vi "Instrumento_caracterizacion_4.vi"() -> ()   [LabVIEW 2013]
uses:
  <vilib>/Analysis/NI_AALBase.lvlib
panel:
  in  "Tab Control":enum32{"Live Picture", "ICImagingControl"}(tab)
  out "Live Picture":picture
  in  "ICImagingControl":refnum<k7>(container)
  in  "Pasos por vuelta\nM1(746)          M2(646)      M3(740)       M4(766)":dbl[](array[numeric])
  in  "Nombre de archivo 2":string="In"
  out "a":bool
  out "Angulo actual":dbl[](array[numeric])
  in  "Ejecutar desde txt":bool
  in  "Txt con medidas a realizar":path=path "C:/Users/franjas/Documents/rutinas-calibracion-slm/measures.txt"
  in  "Camino a ArduinoSteeper.py":path=path "C:/Users/franjas/Documents/rutinas-calibracion-slm"
  in  "Directorio scripts matlab 2":path=path "C:/Users/franjas/Documents/rutinas-calibracion-slm"
  out "o":bool
  in  "Nombre de archivo":string="In1"
  in  "Start":bool
  in  "Seleción método":bool
  in  "Ángulos de elementos ópticos:\nL2_in        L4_in     L4_out  P__out":dbl[](array[numeric])=[0.0, 0.0, 0.0, 0.0]
  in  "Shutter":bool
  in  "Stop VI":bool
  in  "Amp vs ng":bool
  in  "fas vs ng":bool
  in  "Configurar para franjas":bool
  in  "Exit live":bool
  in  "ContinuousCapture":bool
  in  "File to load":path
  in  "File to save":path
  in  "VCD Properties":bool
  in  "Save properties":bool
  in  "Load properties":bool
  out "Video formats":string[](array[string])
  out "Devices":string[](array[string])
  out "Histogram Graph":T1(graph)
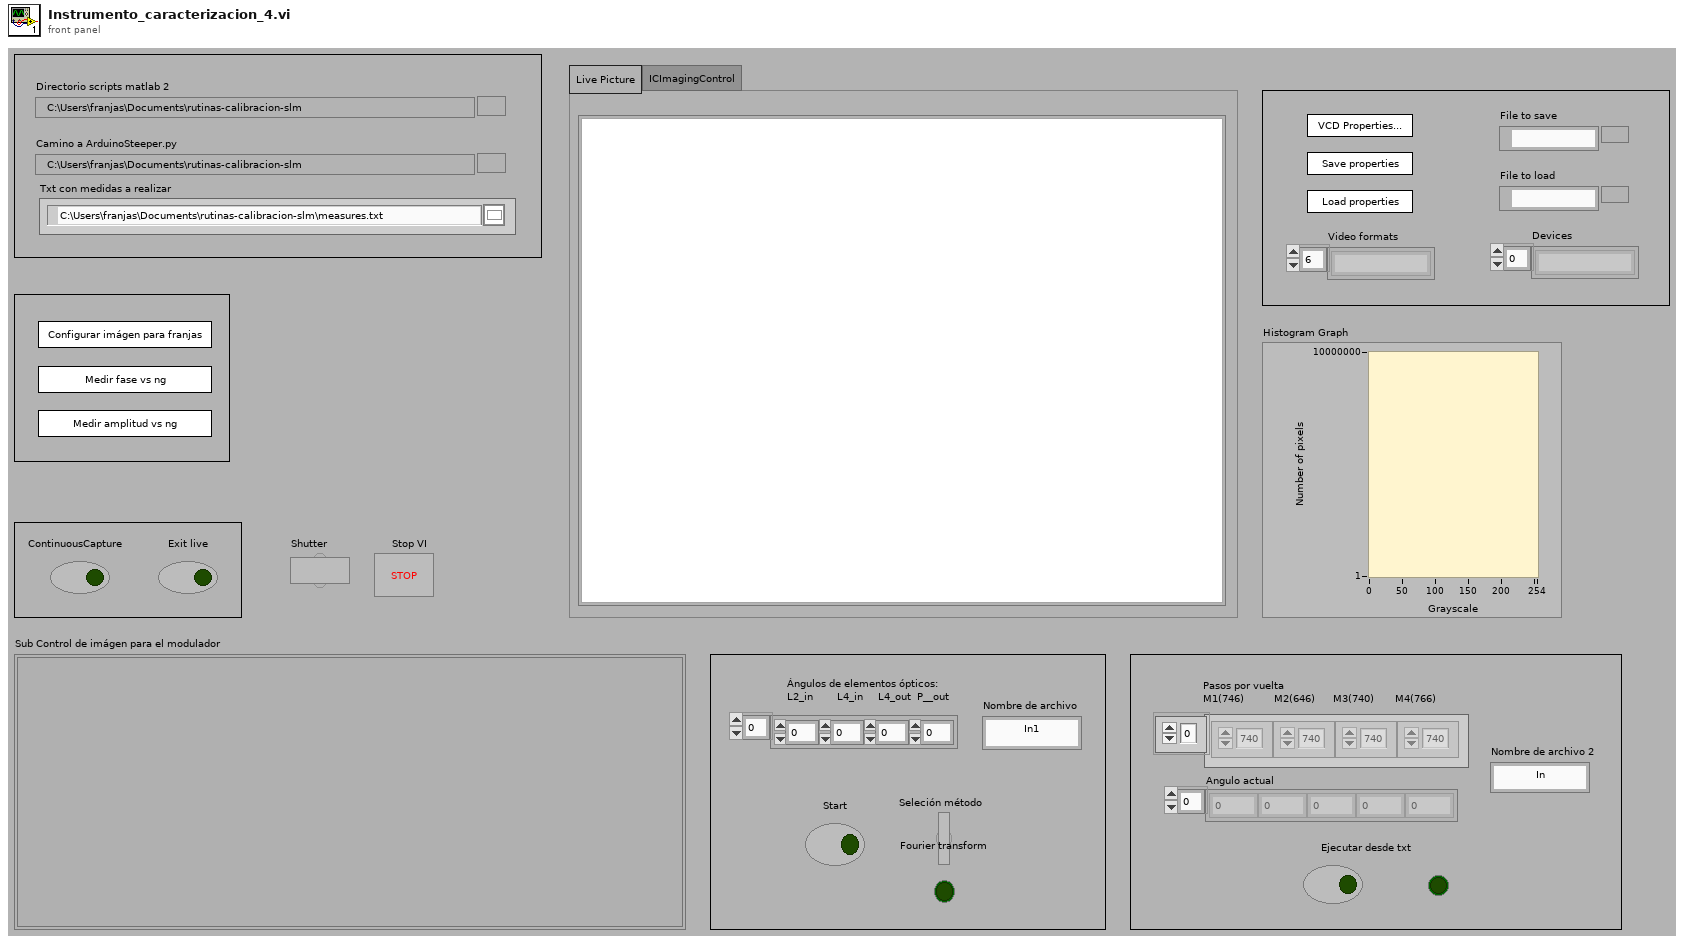
[diagram p1: front panel]
types:
  T1 = cluster{"X Values":dbl[], "Histogram: h(x)":i32[]}
  T2 = typedef "imagedata.ctl" = cluster{"image type":i32, "image depth":i32, "image":u8[], "mask":u8[], "colors":u32[], "Rectangle":cluster{"left":i16, "top":i16, "right":i16, "bottom":i16}}
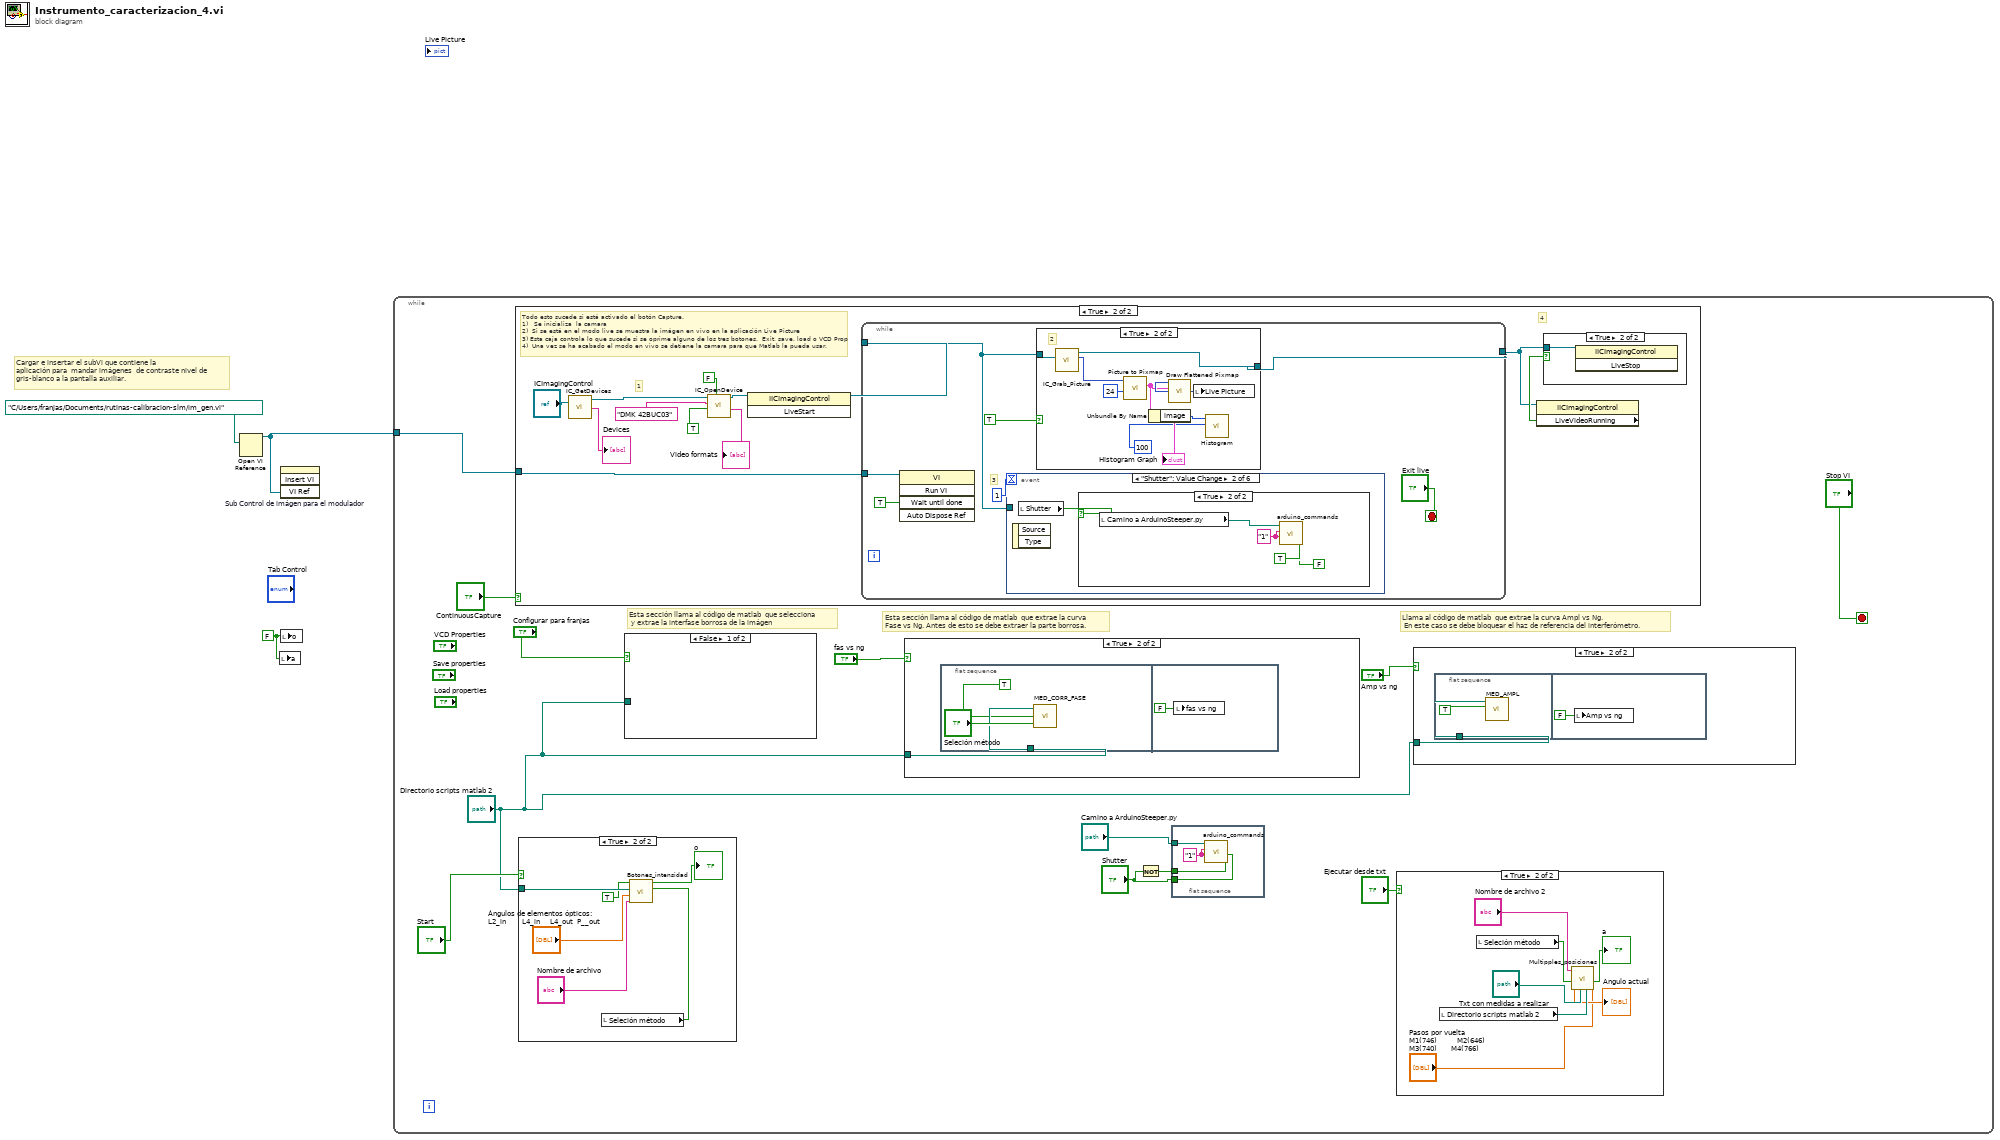
[diagram p0: block diagram]
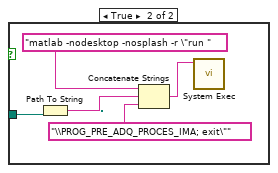
[diagram p6: hidden frame]
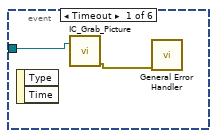
[diagram p8: hidden frame]
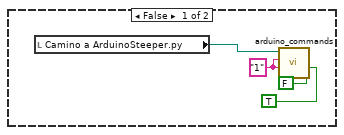
[diagram p9: hidden frame]
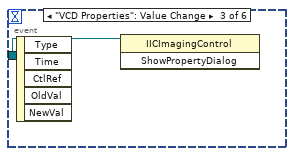
[diagram p10: hidden frame]
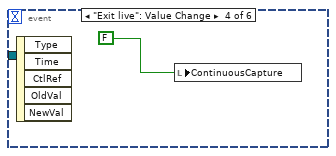
[diagram p11: hidden frame]
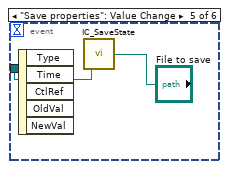
[diagram p12: hidden frame]
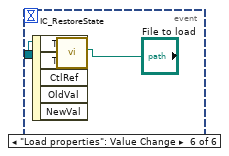
[diagram p13: hidden frame]
diagram:
  w1 = FALSE ("o")
  # "Cargar e insertar el subVi que contiene la \naplicación para  mandar imágenes  de contraste nivel de gris-blanco a la pantalla auxiliar."
  n1 = Open VI Reference(vi path=path "C:/Users/franjas/Documents/rutinas-calibracion-slm/im_gen.vi") -> (vi reference=w2:refnum<vi>)  [unwired: 5 in, 1 out]
  n2 = local write "a"(w1) -> ()
  n3 = invoke on="Sub Control de imágen para el modulador" class="SubPanel" method="Insert VI"("VI Ref"=w2) -> ()  [unwired: 3 in, 4 out]
  n4 = local write "o"(w1) -> ()
  n5 = while {
    tunnel: w2 -> [w13]
    stop <- "Stop VI" stop-if-true
    # "Llama al código de matlab  que extrae la curva Ampl vs Ng.\n En este caso se debe bloquear el haz de referencia del interferómetro."
    # "Esta sección llama al código de matlab  que extrae la curva\nFase vs Ng. Antes de esto se debe extraer la parte borrosa."
    # "Esta sección llama al código de matlab  que selecciona\n y extrae la interfase borrosa de la imágen"
    n6 = case shown="True" "ContinuousCapture" {
      tunnel: w13 -> [_ w47]
      frame False {
      }
      frame True {
        # "4"
        # "1"
        # "Todo esto sucede si está activado el botón Capture.  \n1)   Se inicializa  la camara \n2)  Si se está en el modo live se muestra la imágen en vivo en la aplicación Live Picture\n3) Esta caja controla lo que sucede si se oprime alguno de los tres botones,  Exit, save, load o VCD Prop\n4)  Una vez se ha acabado el modo en vivo se detiene la camara para que Matlab la pueda usar."
        n7 = call <userlib>:"IC_GetDevices.vi"("ICImagingControl In"="ICImagingControl") -> ("ICImagingControl Out"=w56:refnum<k7>, "Devices"=→"Devices":string[])  [unwired: 1 in, 1 out]
        n8 = call <userlib>:"IC_OpenDevice.vi"("Color"=FALSE, "Live"=TRUE, "Device"="DMK 42BUC03", "ICImagingControl In"=w56) -> ("VideoFormats"=→"Video formats":string[], "ICImagingControl Out"=w50:refnum<k7>)  [unwired: 2 in, 4 out]
        n9 = invoke class="IICImagingControl" method="LiveStart"(reference=w50) -> (reference out=w48:refnum<k7>)  [unwired: 2 in, 2 out]
        n10 = while {
          tunnel: w48 -> [w62]
          tunnel: [w65] -> w49
          tunnel: w47 -> [w64]
          stop <- "Exit live" stop-if-true
          # "3"
          n11 = invoke class="VI" method="Run VI"(reference=w64, "Wait until done"=TRUE ("Wait Until Done")) -> ()  [unwired: 3 in, 5 out]
          n12 = event shown="[1] \"Shutter\": Value Change" {
            selector: _ -> [_ _ _ _ _ _]
            dyn-events: _ -> [_ _ _ _ _ _]
            timeout: 1 -> [_ _ _ _ _ _]
            tunnel: w62 -> [w66 _ w77 _ w80 w82]
            event Timeout {
              n13 = event-data() -> ()  [unwired: 1 in, 2 out]
              n14 = call <userlib>:"IC_Grab_Picture.vi"("ICImagingControl In"=w66) -> ("Error Out"=w67:errorcluster)  [unwired: 1 in, 3 out]
              n15 = call <vilib>:"General Error Handler.vi"("error in (no error)"=w67) -> ()  [unwired: 10 in, 5 out]
            }
            event "Shutter": Value Change {
              n16 = event-data() -> ()  [unwired: 1 in, 2 out]
              n17 = local read "Shutter"() -> (w68:bool)
              n18 = case shown="True" w68 {
                frame False {
                  w71 = "1" ("Argumento")
                  n19 = local read "Camino a ArduinoSteeper.py"() -> (w72:path)
                  n20 = call "arduino_commands.vi"("Shutter off"=FALSE, "Shutter on"=TRUE ("Shutter off"), "Argumento"=w71, "Número de motor"=w71, "Directorio scripts ArduinoStepper.py"=w72) -> ()  [unwired: 6 in, 1 out]
                }
                frame True {
                  w75 = "1" ("Argumento")
                  n21 = local read "Camino a ArduinoSteeper.py"() -> (w76:path)
                  n22 = call "arduino_commands.vi"("Shutter off"=TRUE, "Shutter on"=FALSE, "Argumento"=w75, "Número de motor"=w75, "Directorio scripts ArduinoStepper.py"=w76) -> ()  [unwired: 6 in, 1 out]
                }
              }
            }
            event "VCD Properties": Value Change {
              n23 = event-data() -> ()  [unwired: 1 in, 5 out]
              n24 = invoke class="IICImagingControl" method="ShowPropertyDialog"(reference=w77) -> ()  [unwired: 2 in, 3 out]
            }
            event "Exit live": Value Change {
              n25 = event-data() -> ()  [unwired: 1 in, 5 out]
              n26 = local write "ContinuousCapture"(FALSE ("CApture")) -> ()
            }
            event "Save properties": Value Change {
              n27 = event-data() -> ()  [unwired: 1 in, 5 out]
              n28 = call <userlib>:"IC_SaveState.vi"("file path"="File to save", "ICImagingControl In"=w80) -> ()  [unwired: 1 in, 2 out]
            }
            event "Load properties": Value Change {
              n29 = event-data() -> ()  [unwired: 1 in, 5 out]
              n30 = call <userlib>:"IC_RestoreState.vi"("File Path"="File to load", "ICImagingControl"=w82) -> ()  [unwired: 2 in, 2 out]
            }
          }
          n31 = case shown="True" TRUE {
            tunnel: w62 -> [w83 w89]
            tunnel: [w83 w84] -> w65
            frame False {
            }
            frame True {
              # "2"
              n32 = call <userlib>:"IC_Grab_Picture.vi"("ICImagingControl In"=w89) -> ("ICImagingControl Out"=w84:refnum<k7>, "Picture Out"=w92:picture)  [unwired: 1 in, 2 out]
              n33 = call <vilib>:"Picture to Pixmap.vi"("depth"=24, "picture"=w92) -> ("image data"=w88:T2)  [unwired: 8 in, 1 out]
              n34 = Unbundle By Name(w88) -> ("image"=w87:u8[])
              n35 = call <vilib>:"Draw Flattened Pixmap.vi"("image data"=w88) -> ("new picture"=w90:picture)  [unwired: 8 in]
              n36 = local write "Live Picture"(w90) -> ()
              n37 = call <vilib>:"Histogram.vi"("intervals"=100, "X"=w87) -> ("Histogram Graph"=→"Histogram Graph":T1)  [unwired: 6 in, 3 out]
            }
          }
        }
        n38 = property class="IICImagingControl"(reference=w49) -> ("LiveVideoRunning"=w51:bool)  [unwired: 1 in, 2 out]
        n39 = case shown="True" w51 {
          tunnel: w49 -> [_ w93]
          frame False {
          }
          frame True {
            n40 = invoke class="IICImagingControl" method="LiveStop"(reference=w93) -> ()  [unwired: 2 in, 3 out]
          }
        }
      }
    }
    n41 = case shown="True" "Start" {
      tunnel: "Directorio scripts matlab 2" -> [_ w32]
      frame False {
      }
      frame True {
        n42 = local read "Seleción método"() -> (w29:bool)
        n43 = call "Botones_intensidad.vi"("Seleción método"=w29, "String"="Nombre de archivo", "Array"="Ángulos de elementos ópticos:\nL2_in        L4_in     L4_out  P__out", "Directorio scripts matlab 2"=w32, "I1"=TRUE) -> (3:→"o":bool)  [unwired: 6 in]
      }
    }
    n44 = case shown="False" "Configurar para franjas" {
      tunnel: "Directorio scripts matlab 2" -> [_ w42]
      frame False {
      }
      frame True {
        n45 = Path To String(path=w42) -> (string=w46:string)
        n46 = Concatenate Strings("matlab -nodesktop -nosplash -r \"run " ("command line"), w46, "\\PROG_PRE_ADQ_PROCES_IMA; exit\"" ("command line")) -> (w45:string)
        n47 = call <vilib>:"System Exec.vi"("command line"=w45) -> ()  [unwired: 7 in, 4 out]
      }
    }
    n48 = case shown="True" "fas vs ng" {
      tunnel: "Directorio scripts matlab 2" -> [_ w37]
      frame False {
      }
      frame True {
        n49 = flat-sequence {
          tunnel: w37 -> [w39]
          frame #0 {
            n50 = call "MED_CORR_FASE.vi"("Seleción método"="Seleción método", "Ejecucion"=TRUE ("Boolean"), "Directorio scripts matlab"=w39) -> ()
          }
          frame #1 {
            n51 = local write "fas vs ng"(FALSE ("fas vs ng")) -> ()
          }
        }
      }
    }
    n52 = Not(x="Shutter") -> (.not. x?=w6:bool)
    n53 = flat-sequence {
      tunnel: "Camino a ArduinoSteeper.py" -> [w26]
      tunnel: w6 -> [w25]
      tunnel: "Shutter" -> [w24]
      frame #0 {
        w23 = "1" ("Argumento")
        n54 = call "arduino_commands.vi"("Shutter off"=w25, "Shutter on"=w24, "Argumento"=w23, "Número de motor"=w23, "Directorio scripts ArduinoStepper.py"=w26) -> ()  [unwired: 6 in, 1 out]
      }
    }
    n55 = case shown="True" "Ejecutar desde txt" {
      frame False {
      }
      frame True {
        n56 = local read "Directorio scripts matlab 2"() -> (w21:path)
        n57 = local read "Seleción método"() -> (w19:bool)
        n58 = call "Multipples_posiciones.vi"("Pasos por vuelta\nM1                 M2              M3            M4"="Pasos por vuelta\nM1(746)          M2(646)      M3(740)       M4(766)", "Directorio scripts matlab 2"=w21, "File Path Control"="Txt con medidas a realizar", "Seleción método"=w19, "Nombre de archivo 2"="Nombre de archivo 2") -> (1:→"a":bool, "subarray"=→"Angulo actual":dbl[])  [unwired: 5 in]
      }
    }
    n59 = case shown="True" "Amp vs ng" {
      tunnel: "Directorio scripts matlab 2" -> [_ w33]
      frame False {
      }
      frame True {
        n60 = flat-sequence {
          tunnel: w33 -> [w35]
          frame #0 {
            n61 = call "MED_AMPL.vi"("Boolean"=TRUE, "Directorio scripts matlab"=w35) -> ()  [unwired: 10 in]
          }
          frame #1 {
            n62 = local write "Amp vs ng"(FALSE ("Amp vs ng")) -> ()
          }
        }
      }
    }
  }
